vi "Main.vi"() -> ()   [LabVIEW 2016]
doc: "This template is for the Queued Message Handler design pattern.\n\nThe Event Handling Loop generates messages based on user interface actions.\n\nThe Message Handling Loop processes messages generated by the Event Handling Loop, or by other messages. The messages are string values, so new messages can be added easily to the Message Cases case structure in the Message Handling Loop. Each message cluster can also provide an optional value for Message Data, which is a variant that can be converted to whatever message-specific data is required."
uses:
  controls/UI Data.ctl
  support/Message Queue/Message Queue.lvlib
  <vilib>/Utility/error.llb/Error Cluster From Error Code.vi
  support/User Event - Stop/User Event - Stop.lvlib
  support/Message Queue/Enqueue Message (Single).vi
  <vilib>/ErrorRing/Error Ring.xnode
  <vilib>/SmarAct/MCS/Types/mcsSensorTypes.ctl
  helper/revolution_parameters.ctl
panel:
  in  "revolution":i32
  in  "Init Stages":bool
  out "stepsize y":dbl
  out "stepsize x":dbl
  in  "Iteration":u32=1
  in  "RESET PREV RUN":bool
  in  "ABORT":bool
  in  "RUN TABLE":bool
  in  "Angle":i32=16960
  in  "DISTANCE Y":i32=16960
  in  "one revolution":bool
  in  "steps Y":i32
  in  "scan length y (micron)":dbl format="%#_13g"
  out "polling iteration":i32=3
  in  "System locator":string(combo)="usb:id:425839965"
  in  "findSystems":bool caption="Find Systems"
  out "hw loop current msg":string="Exit"
  in  "init loops test":bool
  in  "stop":bool
  in  "DISTANCE X":i32=16960
  in  "one step y":bool
  in  "one step x":bool
  out "channelIndex":u32
  out "data1 2":u32=143
  out "packetType":T1(ring)=enum."SA_ERROR_ PACKET_TYPE"
  in  "connect":bool
  out "connected":bool=TRUE
  in  "Amplitude":u32=4000 min=1 max=4000 step=1
  in  "Frequency":u32=8000 min=1 max=18500 step=1
  in  "Rotation channel":u32
  in  "Y channel":u32=2
  out "Error":errorcluster
  in  "X channel":u32=1
  out "System Index":u32=35
  out "Y array":dbl[](array[numeric])
  out "X array":dbl[](array[numeric])
  in  "scan length x (micron)":dbl format="%#_13g"
  in  "steps X":i32
  in  "calc table":bool=TRUE
  in  "Home":bool
  out "Display <Replace Me>":string="\"Exit\" button pressed"
  in  "Do Something Else <Replace Me>":bool
  in  "Do Something <Replace Me>":bool
  in  "Exit":bool
  # "These controls have associated \"Value Changed\" events configured in the Event Structure on the diagram.\n\nReplace them (and reconfigure the Event Structure) with the controls you need for your application."
  # "This template is for the Queued Message Handler design pattern.\n\nSee the block diagram for more information on how to use this template."
  # "POLLING"
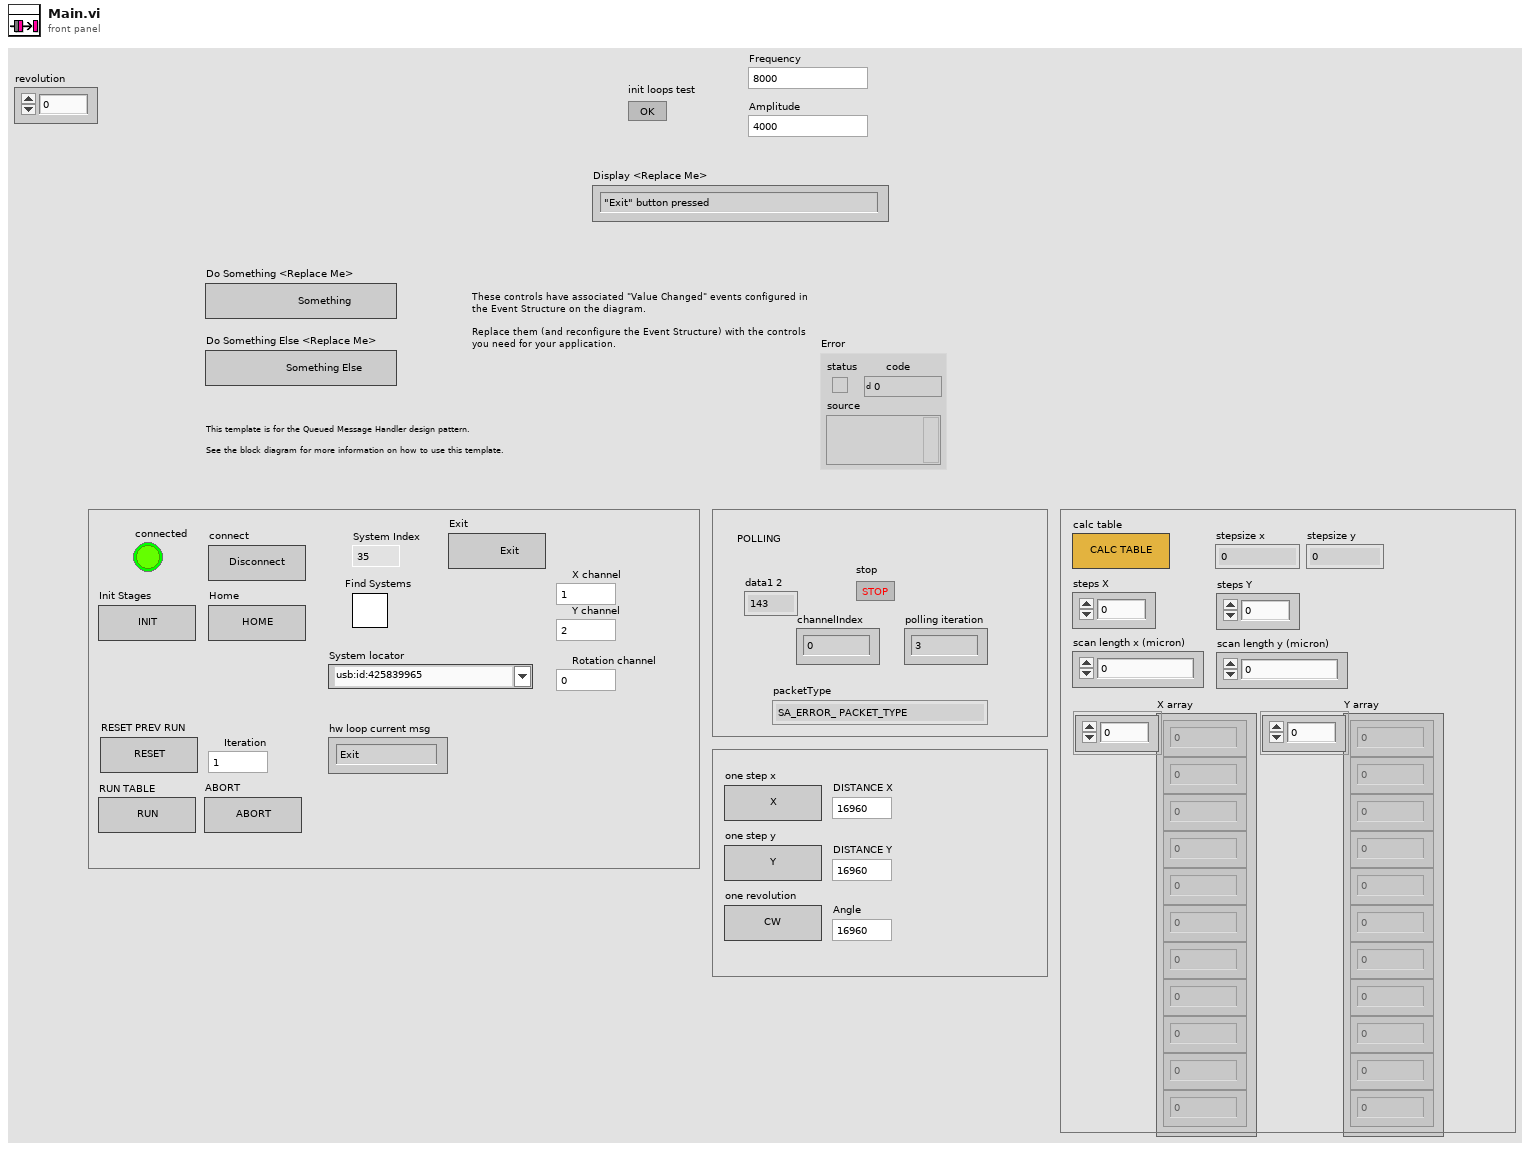
[diagram p1: front panel]
types:
  T1 = enum32{"SA_NO PACKET_TYPE", "SA_ERROR_ PACKET_TYPE", "SA_POSITION PACKET_TYPE", "SA_COMPLETED PACKET_TYPE", "SA_STATUS PACKET_TYPE", "SA_ANGLE_PACKET_TYPE", "SA_VOLTAGE_LEVEL_PACKET_TYPE", "SA_SENSOR_TYPE_PACKET_TYPE", "SA_SENSOR_ENABLED_PACKET_TYPE", "SA_END_EFFECTOR_TYPE_PACKET_TYPE", "SA_GRIPPER_OPENING_PACKET_TYPE", "SA_FORCE_PACKET_TYPE", "SA_MOVE_SPEED_PACKET_TYPE", "SA_PHYSICAL_POSITION_KNOWN_PACKET_TYPE", "SA_POSITION_LIMIT_PACKET_TYPE", "SA_ANGLE_LIMIT_PACKET_TYPE", "SA_SAFE_DIRECTION_PACKET_TYPE", "SA_SCALE_PACKET_TYPE", "SA_MOVE_ACCELERATION_PACKET_TYPE", "SA_CHANNEL_PROPERTY_PACKET_TYPE", "SA_CAPTURE_BUFFER_PACKET_TYPE", "SA_TRIGGERED_PACKET_TYPE"}
  T2 = typedef "UI Data.ctl" = cluster{"Boolean <Replace Me>":bool, "String <Replace Me>":string, "Numeric <Replace Me>":dbl, "Do Something Ref":refnum<vi>, "Do Something Else Ref":refnum<vi>, "Data Display Ref":refnum<vi>, "Exit Button Ref":refnum<vi>}
  T3 = typedef "Message Queue.lvlib/All Message Queues.ctl" = cluster{"UI":refnum<queue>, "queue out":refnum<queue>}
  T4 = typedef "mcsSensorTypes.ctl" = enum32{"SA_NO_SENSOR_TYPE", "SA_S_SENSOR_TYPE", "SA_SR_SENSOR_TYPE", "SA_ML_SENSOR_TYPE", "SA_MR_SENSOR_TYPE", "SA_SP_SENSOR_TYPE", "SA_SC_SENSOR_TYPE", "SA_M25_SENSOR_TYPE", "SA_SR20_SENSOR_TYPE", "SA_M_SENSOR_TYPE", "SA_GC_SENSOR_TYPE", "SA_GD_SENSOR_TYPE", "SA_GE_SENSOR_TYPE", "SA_RA_SENSOR_TYPE", "SA_GF_SENSOR_TYPE", "SA_RB_SENSOR_TYPE", "SA_G605S_SENSOR_TYPE", "SA_G775S_SENSOR_TYPE", "SA_SC500_SENSOR_TYPE", "SA_G955S_SENSOR_TYPE", "SA_SR77_SENSOR_TYPE", "SA_SD_SENSOR_TYPE", "SA_R20ME_SENSOR_TYPE", "SA_SR2_SENSOR_TYPE", "SA_SCD_SENSOR_TYPE", "SA_SRC_SENSOR_TYPE", "SA_SR36M_SENSOR_TYPE", "SA_SR36ME_SENSOR_TYPE", "SA_SR50M_SENSOR_TYPE", "SA_SR50ME_SENSOR_TYPE", "SA_G1045S_SENSOR_TYPE", "SA_G1395S_SENSOR_TYPE", "SA_MD_SENSOR_TYPE", "SA_G935M_SENSOR_TYPE", "SA_SHL20_SENSOR_TYPE", "SA_SCT_SENSOR_TYPE", "SA_SR77T_SENSOR_TYPE", "SA_SR120_SENSOR_TYPE", "SA_LC_SENSOR_TYPE", "SA_LR_SENSOR_TYPE", "SA_LCD_SENSOR_TYPE", "SA_L_SENSOR_TYPE", "SA_LD_SENSOR_TYPE", "SA_LE_SENSOR_TYPE", "SA_LED_SENSOR_TYPE", "SA_GDD_SENSOR_TYPE", "SA_GED_SENSOR_TYPE", "SA_G935S_SENSOR_TYPE", "SA_G605DS_SENSOR_TYPE", "SA_G775DS_SENSOR_TYPE"}
  T5 = enum32{"SA_NO_REPORT_ON_COMPLETE", "SA_REPORT_ON_COMPLETE"}
  T6 = enum32{"SA_SENSOR_DISABLED", "SA_SENSOR_ENABLED", "SA_SENSOR_POWERSAVE"}
  T7 = enum32{"SA_UNBUFFERED_OUTPUT", "SA_BUFFERED_OUTPUT"}
  T8 = typedef "revolution_parameters.ctl" = cluster{"revolution":i32, "angle":i32}
  T9 = typedef "mcsPacket.ctl" = cluster{"packetType":enum32{"SA_NO PACKET_TYPE", "SA_ERROR_ PACKET_TYPE", "SA_POSITION PACKET_TYPE", "SA_COMPLETED PACKET_TYPE", "SA_STATUS PACKET_TYPE", "SA_ANGLE_PACKET_TYPE", "SA_VOLTAGE_LEVEL_PACKET_TYPE", "SA_SENSOR_TYPE_PACKET_TYPE", "SA_SENSOR_ENABLED_PACKET_TYPE", "SA_END_EFFECTOR_TYPE_PACKET_TYPE", "SA_GRIPPER_OPENING_PACKET_TYPE", "SA_FORCE_PACKET_TYPE", "SA_MOVE_SPEED_PACKET_TYPE", "SA_PHYSICAL_POSITION_KNOWN_PACKET_TYPE", "SA_POSITION_LIMIT_PACKET_TYPE", "SA_ANGLE_LIMIT_PACKET_TYPE", "SA_SAFE_DIRECTION_PACKET_TYPE", "SA_SCALE_PACKET_TYPE", "SA_MOVE_ACCELERATION_PACKET_TYPE", "SA_CHANNEL_PROPERTY_PACKET_TYPE", "SA_CAPTURE_BUFFER_PACKET_TYPE", "SA_TRIGGERED_PACKET_TYPE"}, "channelIndex":u32, "data1":u32, "data2":i32, "data3":i32, "data4":u32}
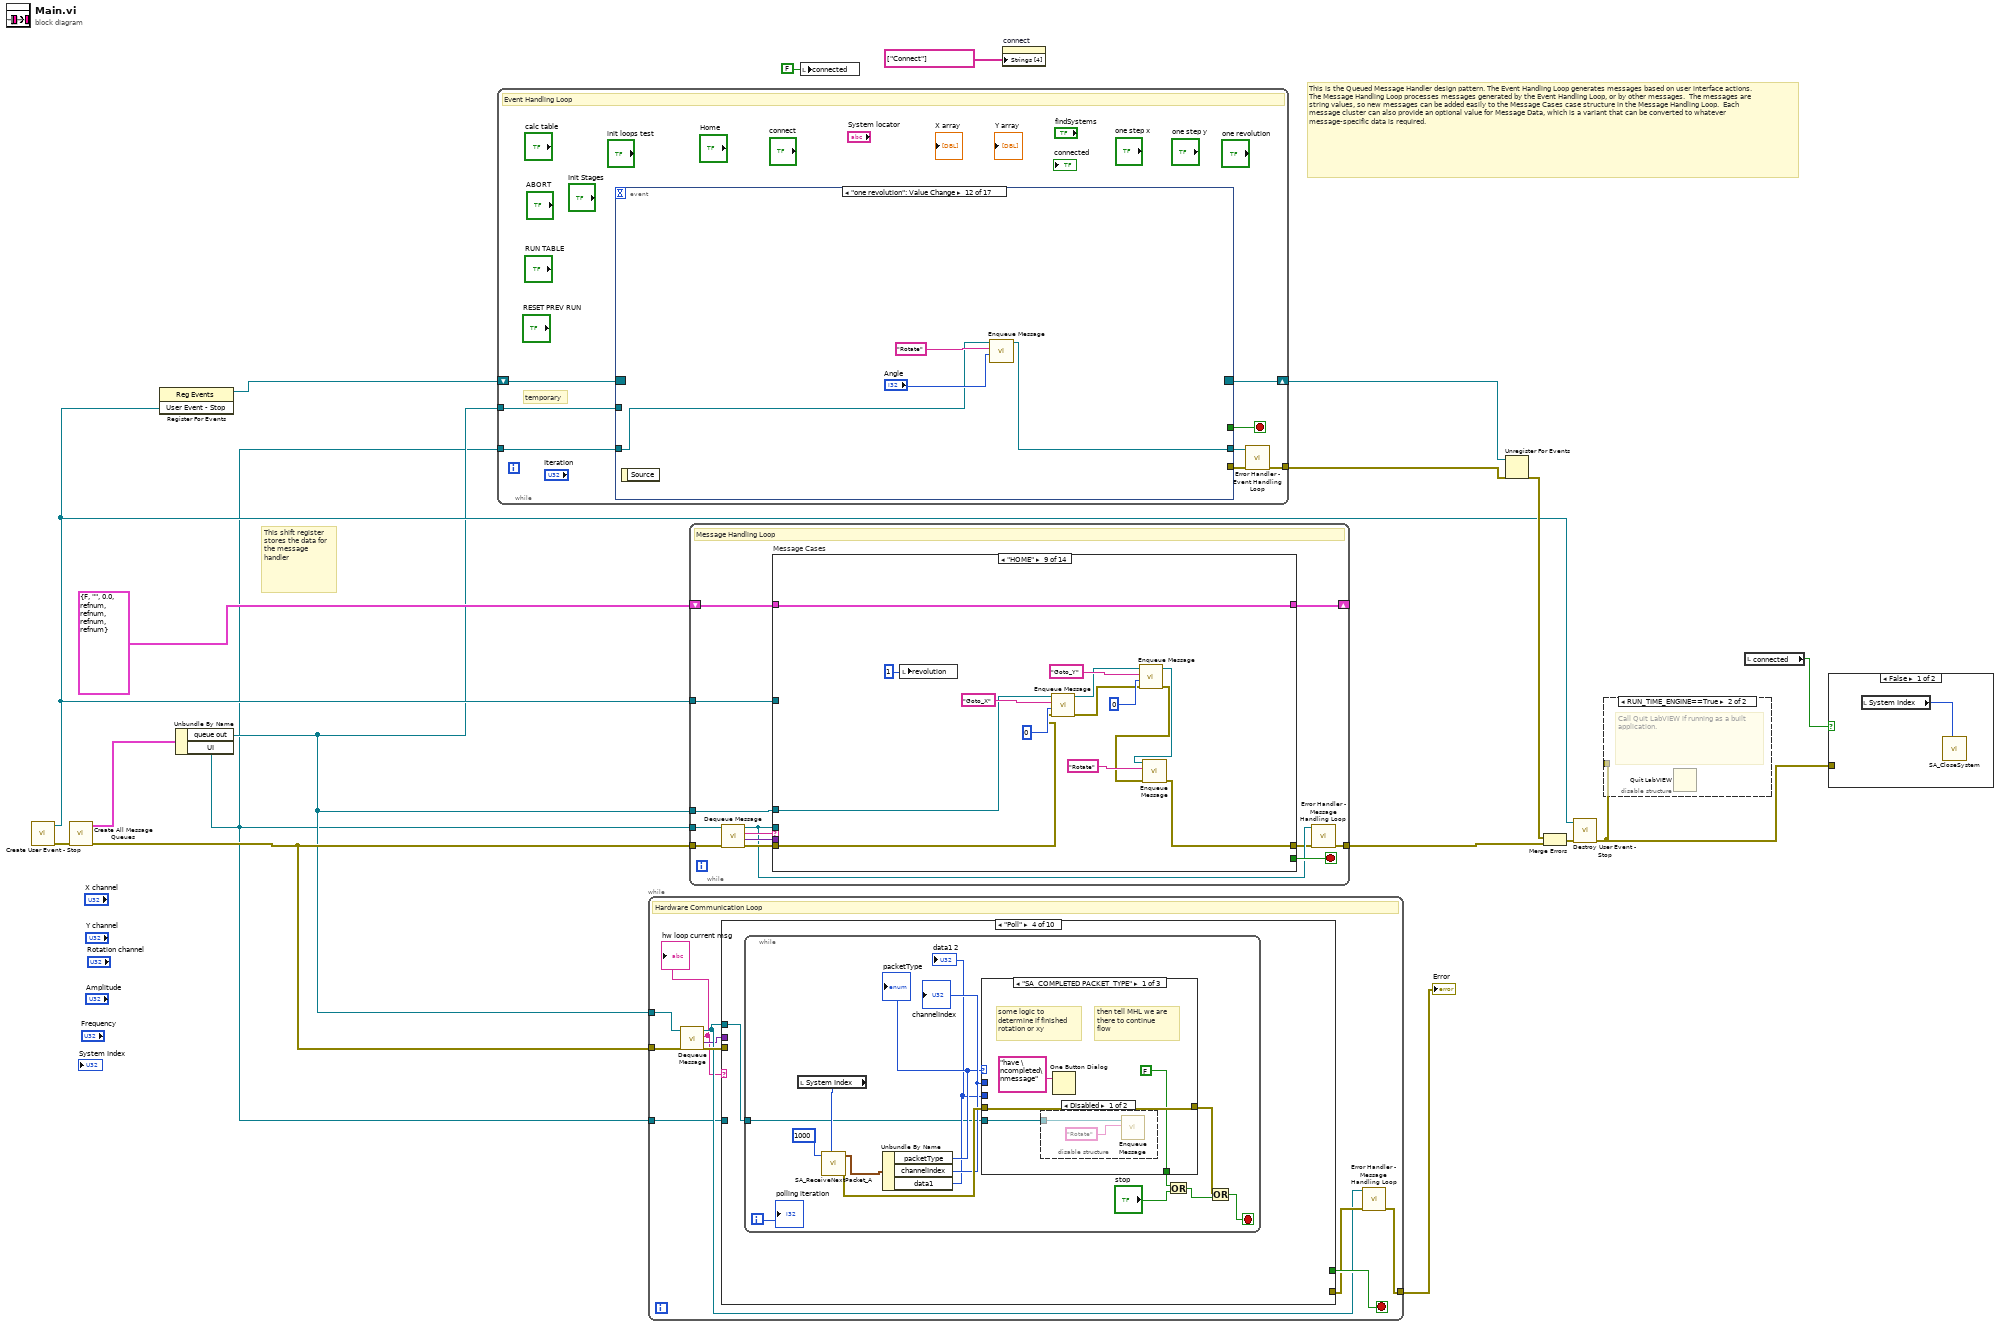
[diagram p0: block diagram]
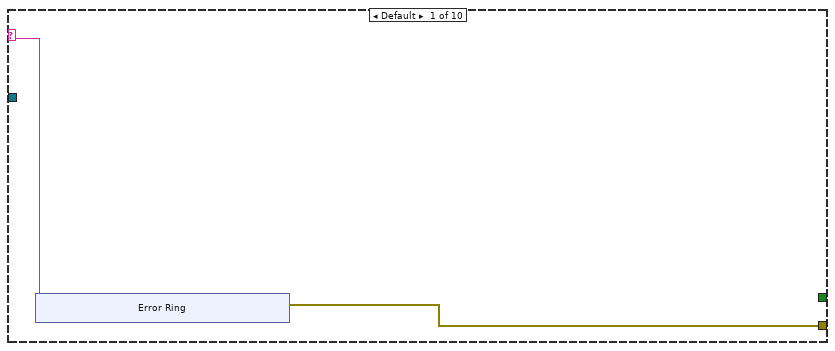
[diagram p3: hidden frame]
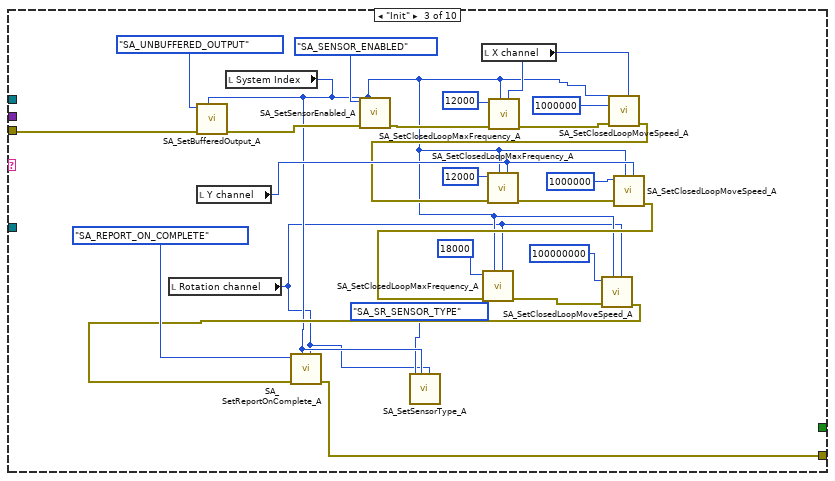
[diagram p5: hidden frame]
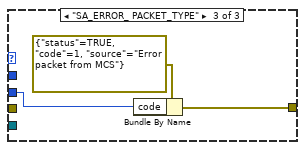
[diagram p8: hidden frame]
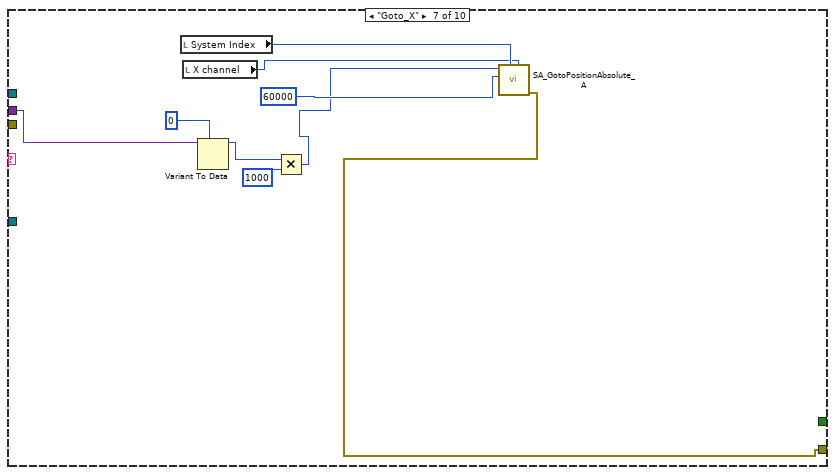
[diagram p11: hidden frame]
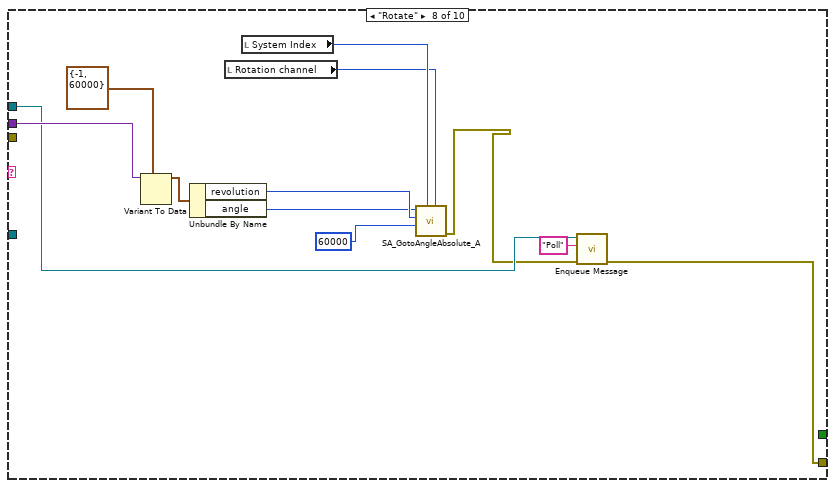
[diagram p12: hidden frame]
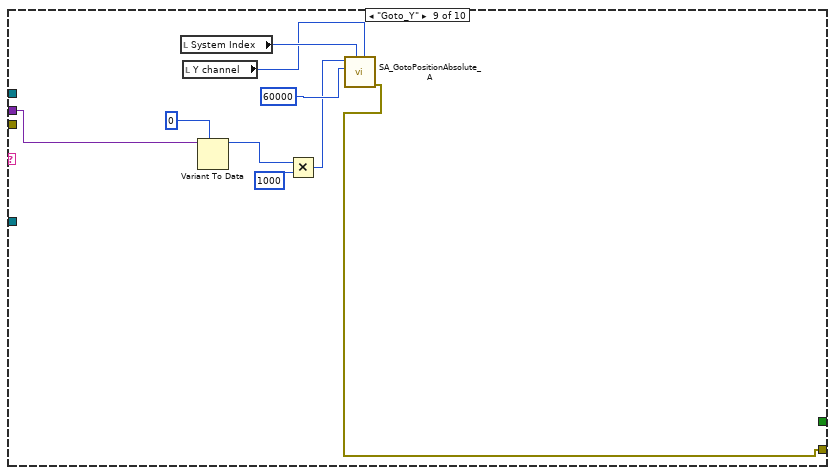
[diagram p13: hidden frame]
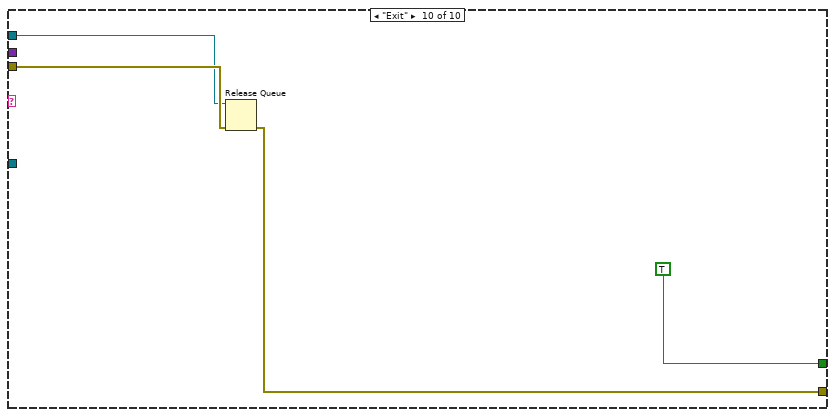
[diagram p14: hidden frame]
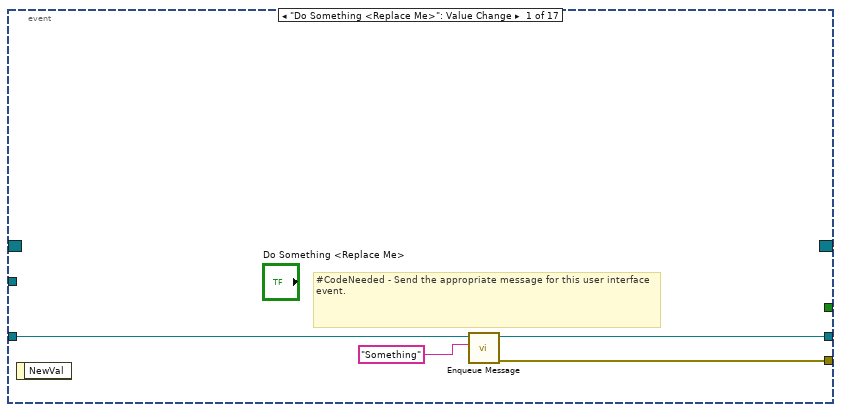
[diagram p16: hidden frame]
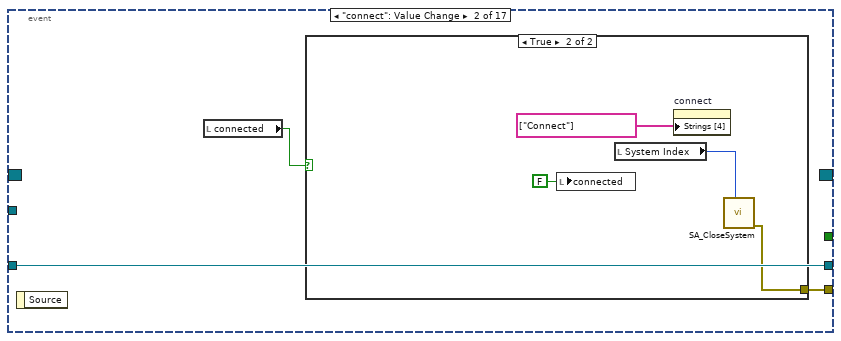
[diagram p17: hidden frame]
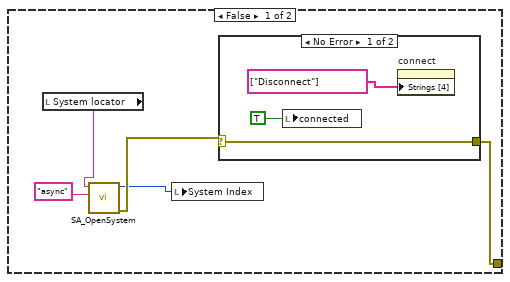
[diagram p18: hidden frame]
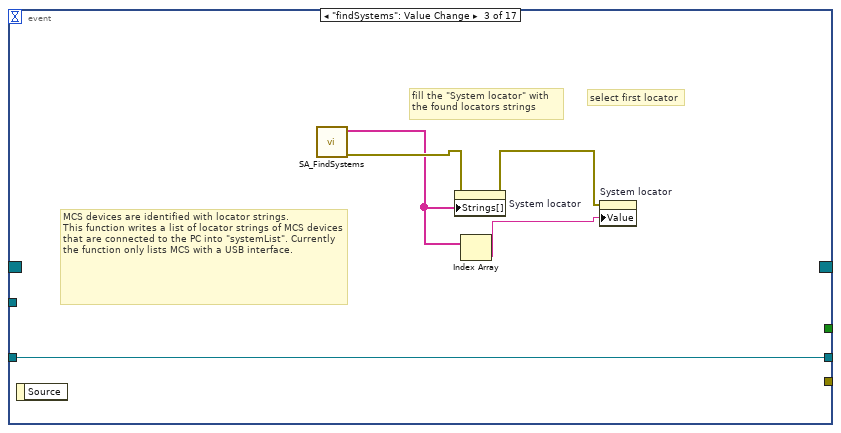
[diagram p20: hidden frame]
diagram:
  # "This is the Queued Message Handler design pattern. The Event Handling Loop generates messages based on user interface actions. The Message Handling Loop processes messages generated by the Event Handling Loop, or by other messages.  The messages are string values, so new messages can be added easily to the Message Cases case structure in the Message Handling Loop.  Each message cluster can also provide an optional value for Message Data, which is a variant that can be converted to whatever message-specific data is required."
  # "This shift register stores the data for the message handler"
  n1 = call "Create User Event - Stop.vi"() -> ("error out"=w16:errorcluster, "User Event - Stop"=w9:refnum<user-event>)  [unwired: 10 in]
  n2 = call "Create All Message Queues.vi"("error in (no error)"=w16) -> ("error out"=w7:errorcluster, "Message Queues out"=w18:T3)  [unwired: 9 in]
  n3 = register-events(w9) -> (reference out=w10:refnum<event-registration>)  [unwired: 2 in, 1 out]
  n4 = Unbundle By Name(w18) -> ("queue out"=w2:refnum<queue>, "UI"=w1:refnum<queue>)
  n5 = while {
    tunnel: w1 -> [w26]
    shift-right: [w24] -> w13
    shift-left: w10 -> [w25]
    tunnel: [w20] -> w11
    tunnel: w2 -> [w19]
    stop <- w22 stop-if-true
    # "temporary"
    # "Event Handling Loop"
    n6 = event shown="[11] \"one revolution\": Value Change" {
      selector: w25 -> [_ _ _ _ _ _ _ _ _ _ _ _ _ _ _ _ _]
      dyn-events: [_ _ _ _ _ _ _ _ _ _ _ _ _ _ _ _ _] -> w24
      timeout: _ -> [_ _ _ _ _ _ _ _ _ _ _ _ _ _ _ _ _]
      tunnel: [_ _ _ _ _ _ _ _ _ _ _ _ _ _ _ _ TRUE ("Discard?")] -> w22
      tunnel: w26 -> [w30 w33 w51 w55 w57 w66 w70 w72 w77 w78 w83 w87 w93 w98 w100 w105 w108]
      tunnel: [w27 w32 _ w52 _ _ w68 _ w75 _ _ _ w90 w97 _ w104 _] -> w23
      tunnel: [w29 w33 w51 w54 w57 w66 w69 w71 w76 w78 w83 w86 w92 w96 w100 w103 w108] -> w21
      tunnel: w19 -> [_ _ _ _ _ _ _ _ _ w79 w84 _ _ _ _ _ _]
      event "Do Something <Replace Me>": Value Change {
        # "#CodeNeeded - Send the appropriate message for this user interface event."
        n7 = event-data() -> ()  [unwired: 1 in, 1 out]
        n8 = call-poly "Enqueue Message.vi"("Message"="Something", "Message Queue"=w30) -> ("error out"=w27:errorcluster, "dup Message Queue"=w29:refnum<queue>)  [unwired: 8 in]
      }
      event "connect": Value Change {
        n9 = event-data() -> ()  [unwired: 1 in, 1 out]
        n10 = local read "connected"() -> (w31:bool)
        n11 = case shown="True" w31 {
          tunnel: [w36 w43] -> w32
          frame False {
            n12 = local read "System locator"() -> (w35:string)
            n13 = call <vilib>:"SA_OpenSystem.vi"("options"="async", "systemLocator"=w35) -> ("error out"=w37:errorcluster, "systemIndexOut"=w34:u32)  [unwired: 8 in]
            n14 = local write "System Index"(w34) -> ()
            n15 = case shown="No Error" w37 {
              selector: w37 -> [w40 w42]
              tunnel: [w40 w42] -> w36
              frame No Error {
                n16 = local write "connected"(TRUE ("connected")) -> ()
                n17 = property on="connect" class="Bool"("Strings [4]"=string[] ["Disconnect"]) -> ()  [unwired: 2 in, 2 out]
              }
              frame Error {
              }
            }
          }
          frame True {
            n18 = local write "connected"(FALSE ("connected")) -> ()
            n19 = local read "System Index"() -> (w44:u32)
            n20 = property on="connect" class="Bool"("Strings [4]"=string[] ["Connect"]) -> ()  [unwired: 2 in, 2 out]
            n21 = call <vilib>:"SA_CloseSystem.vi"("systemIndex"=w44) -> ("error out"=w43:errorcluster)  [unwired: 10 in]
          }
        }
      }
      event "findSystems": Value Change {
        # "select first locator"
        # "fill the \"System locator\" with\nthe found locators strings"
        # "MCS devices are identified with locator strings.\nThis function writes a list of locator strings of MCS devices that are connected to the PC into \"systemList\". Currently the function only lists MCS with a USB interface."
        n22 = event-data() -> ()  [unwired: 1 in, 1 out]
        n23 = call <vilib>:"SA_FindSystems.vi"() -> ("error out"=w50:errorcluster, "systemList"=w49:string[])  [unwired: 10 in]
        n24 = property on="System locator" class="CmbBox"(error in=w50, "Strings[]"=w49) -> (error out=w48:errorcluster)  [unwired: 1 in, 1 out]
        n25 = Index Array(array=w49) -> (element=w47:string)  [unwired: 1 in]
        n26 = property on="System locator" class="CmbBox"(error in=w48, "Value"=w47) -> ()  [unwired: 1 in, 2 out]
      }
      event "init loops test": Value Change {
        n27 = event-data() -> ()  [unwired: 1 in, 1 out]
        n28 = call-poly "Enqueue Message.vi"("Message"="initialize", "Message Queue"=w55) -> ("error out"=w52:errorcluster, "dup Message Queue"=w54:refnum<queue>)  [unwired: 8 in]
      }
      event "RESET PREV RUN": Value Change {
        n29 = event-data() -> ()  [unwired: 1 in, 1 out]
        n30 = local write "Iteration"(u32 0 ("Iteration")) -> ()
      }
      event "calc table": Value Change {
        # "these are both 1D arrays \nof length stepsx * stepsy\nessentially lookup tables"
        n31 = event-data() -> ()  [unwired: 1 in, 1 out]
        n32 = call "calculateTableSimpleSerpentine.vi"("scan length y"="scan length y (micron)", "steps Y"="steps Y", "scan length x"="scan length x (micron)", "steps X"="steps X") -> ("stepsize y"=→"stepsize y":dbl, "final array Y"=w60:dbl[], "stepsize x"=→"stepsize x":dbl, "final array X"=w61:dbl[])
        n33 = local write "Y array"(w60) -> ()
        n34 = local write "X array"(w61) -> ()
      }
      event "Home": Value Change {
        n35 = event-data() -> ()  [unwired: 1 in, 1 out]
        n36 = call-poly "Enqueue Message.vi"("Message"="HOME", "Message Queue"=w70) -> ("error out"=w68:errorcluster, "dup Message Queue"=w69:refnum<queue>)  [unwired: 8 in]
      }
      event "Init Stages": Value Change {
        n37 = event-data() -> ()  [unwired: 1 in, 1 out]
        n38 = call-poly "Enqueue Message.vi"("Message"="START", "Message Queue"=w72) -> ("dup Message Queue"=w71:refnum<queue>)  [unwired: 8 in, 1 out]
      }
      event "RUN TABLE": Value Change {
        n39 = event-data() -> ()  [unwired: 1 in, 1 out]
        n40 = call-poly "Enqueue Message.vi"("Message"="Move_XY", "Message Queue"=w77) -> ("error out"=w75:errorcluster, "dup Message Queue"=w76:refnum<queue>)  [unwired: 8 in]
      }
      event "one step x": Value Change {
        n41 = event-data() -> ()  [unwired: 1 in, 1 out]
        n42 = call-poly "Enqueue Message.vi"("Message Data"="DISTANCE X", "Message"="Goto_X", "Message Queue"=w79) -> ()  [unwired: 7 in, 2 out]
      }
      event "one step y": Value Change {
        n43 = event-data() -> ()  [unwired: 1 in, 1 out]
        n44 = call-poly "Enqueue Message.vi"("Message Data"="DISTANCE Y", "Message"="Goto_Y", "Message Queue"=w84) -> ()  [unwired: 7 in, 2 out]
      }
      event "one revolution": Value Change {
        n45 = event-data() -> ()  [unwired: 1 in, 1 out]
        n46 = call-poly "Enqueue Message.vi"("Message Data"="Angle", "Message"="Rotate", "Message Queue"=w87) -> ("dup Message Queue"=w86:refnum<queue>)  [unwired: 7 in, 1 out]
      }
      event "Do Something Else <Replace Me>": Value Change {
        # "#CodeNeeded - Send the appropriate message for this user interface event."
        n47 = event-data() -> ()  [unwired: 1 in, 1 out]
        n48 = call-poly "Enqueue Message.vi"("Message"="Something Else", "Message Queue"=w93) -> ("error out"=w90:errorcluster, "dup Message Queue"=w92:refnum<queue>)  [unwired: 8 in]
      }
      event Panel Close? {
        # "Send the 'Confirm Quit' message if the user closes the panel of the VI. Discard the event so the 'Confirm Quit' message has a chance to run."
        n49 = event-data() -> ()  [unwired: 1 in, 1 out]
        n50 = call-poly "Enqueue Message.vi"("Priority Message? (F)"=TRUE, "Message"="Confirm Quit", "Message Queue"=w98) -> ("error out"=w97:errorcluster, "dup Message Queue"=w96:refnum<queue>)  [unwired: 7 in]
        n51 = event-data("Discard?"=TRUE) -> ()  [unwired: 1 in, 1 out]
      }
      event Application Instance Close {
        # "#CodeRecommended - When a project closes, all VIs within that project are aborted and leave memory. However, any code placed in this event frame is guaranteed to run to completion, so add any cleanup code that absolutely must happen here."
        n52 = event-data() -> ()  [unwired: 1 in, 1 out]
      }
      event "Exit": Value Change {
        n53 = event-data() -> ()  [unwired: 1 in, 1 out]
        n54 = call-poly "Enqueue Message.vi"("Priority Message? (F)"=TRUE, "Message"="Exit", "Message Queue"=w105) -> ("error out"=w104:errorcluster, "dup Message Queue"=w103:refnum<queue>)  [unwired: 7 in]
      }
      event User Event {
        # "The Message Handling Loop processed an \"Exit\" message, which fired this event to stop the Event Handling Loop."
        n55 = event-data() -> ()  [unwired: 1 in, 1 out]
        n56 = local write "Display <Replace Me>"("\"Exit\" button pressed" ("VI Stopped")) -> ()
      }
    }
    n57 = call "Error Handler - Event Handling Loop.vi"("error in (no error)"=w23, "Message Queue"=w21) -> ("dup error in"=w20:errorcluster)  [unwired: 8 in, 1 out]
  }
  n58 = while {
    tunnel: w2 -> [w118]
    tunnel: [w114] -> w8
    tunnel: w7 -> [w111]
    tunnel: w1 -> [w109]
    stop <- w117 stop-if-true
    # "Hardware Communication Loop"
    n59 = call "Dequeue Message.vi"("error in (no error)"=w111, "Message Queue"=w118) -> ("error out"=w116:errorcluster, "Message Data"=w112:variant, "Message"=w110:string, "dup Message Queue"=w113:refnum<queue>)  [unwired: 6 in]
    "hw loop current msg" <- w110
    n60 = case shown="\"Poll\"" w110 {
      selector: w110 -> [w120 _ _ _ _ _ _ _ _ _]
      tunnel: [w119 _ w131 _ _ _ w180 w186 w204 w208] -> w115
      tunnel: [_ _ _ _ _ _ _ _ _ TRUE] -> w117
      tunnel: w116 -> [_ _ w135 _ _ _ _ _ _ w209]
      tunnel: w113 -> [_ _ _ w152 _ _ _ w189 _ w207]
      tunnel: w112 -> [_ _ _ _ _ _ w184 w197 w205 _]
      tunnel: w109 -> [_ _ _ _ _ _ _ _ _ _]
      frame Default {
        n61 = xnode "Error Ring"("parameter 0"=w120) -> ("error out"=w119:errorcluster)
      }
      frame "Initialize" {
      }
      frame "Init" {
        n62 = local read "Rotation channel"() -> (w128:u32)
        n63 = local read "Y channel"() -> (w140:u32)
        n64 = local read "System Index"() -> (w130:u32)
        n65 = call <vilib>:"SA_SetBufferedOutput_A.vi"("systemIndex"=w130, "error in (no error)"=w135, "mode"=T7."SA_UNBUFFERED_OUTPUT") -> ("error out"=w136:errorcluster)  [unwired: 8 in]
        n66 = call <vilib>:"SA_SetSensorEnabled_A.vi"("systemIndex"=w130, "error in (no error)"=w136, "enabled"=T6."SA_SENSOR_ENABLED") -> ("error out"=w139:errorcluster)  [unwired: 8 in]
        n67 = call <vilib>:"SA_SetSensorType_A.vi"("channelIndex"=w128, "systemIndex"=w130, "type"=mcsSensorTypes."SA_SR_SENSOR_TYPE") -> ()  [unwired: 8 in, 1 out]
        n68 = local read "X channel"() -> (w149:u32)
        n69 = call <vilib>:"SA_SetClosedLoopMaxFrequency_A.vi"("channelIndex"=w149, "systemIndex"=w130, "error in (no error)"=w139, "frequency"=u32 12000) -> ("error out"=w147:errorcluster)  [unwired: 7 in]
        n70 = call <vilib>:"SA_SetClosedLoopMoveSpeed_A.vi"("channelIndex"=w149, "systemIndex"=w130, "error in (no error)"=w147, "speed"=u32 1000000) -> ("error out"=w134:errorcluster)  [unwired: 7 in]
        n71 = call <vilib>:"SA_SetClosedLoopMaxFrequency_A.vi"("channelIndex"=w140, "systemIndex"=w130, "error in (no error)"=w134, "frequency"=u32 12000) -> ("error out"=w150:errorcluster)  [unwired: 7 in]
        n72 = call <vilib>:"SA_SetClosedLoopMoveSpeed_A.vi"("channelIndex"=w140, "systemIndex"=w130, "error in (no error)"=w150, "speed"=u32 1000000) -> ("error out"=w133:errorcluster)  [unwired: 7 in]
        n73 = call <vilib>:"SA_SetClosedLoopMaxFrequency_A.vi"("channelIndex"=w128, "systemIndex"=w130, "error in (no error)"=w133, "frequency"=u32 18000) -> ("error out"=w151:errorcluster)  [unwired: 7 in]
        n74 = call <vilib>:"SA_SetClosedLoopMoveSpeed_A.vi"("channelIndex"=w128, "systemIndex"=w130, "error in (no error)"=w151, "speed"=u32 100000000) -> ("error out"=w132:errorcluster)  [unwired: 7 in]
        n75 = call <vilib>:"SA_SetReportOnComplete_A.vi"("channelIndex"=w128, "systemIndex"=w130, "error in (no error)"=w132, "report"=T5."SA_REPORT_ON_COMPLETE") -> ("error out"=w131:errorcluster)  [unwired: 7 in]
      }
      frame "Poll" {
        n76 = while {
          tunnel: w152 -> [w156]
          i -> [w157]
          stop <- w159 stop-if-true
          n77 = local read "System Index"() -> (w161:u32)
          n78 = call <vilib>:"SA_ReceiveNextPacket_A.vi"("systemIndex"=w161, "timeout"=u32 1000) -> ("error out"=w166:errorcluster, "packet"=w163:T9)  [unwired: 8 in]
          n79 = Unbundle By Name(w163) -> ("packetType"=w164:T1, "channelIndex"=w165:u32, "data1"=w160:u32)
          "packetType" <- w164
          "channelIndex" <- w165
          "data1 2" <- w160
          n80 = case shown="\"SA_COMPLETED PACKET_TYPE\"" w164 {
            tunnel: [w170 w173 w175] -> w158
            tunnel: w160 -> [_ _ w174]
            tunnel: w165 -> [_ _ _]
            tunnel: w166 -> [w170 w173 _]
            tunnel: w156 -> [w168 _ _]
            tunnel: [FALSE ("x") _ _] -> w153
            frame "SA_COMPLETED PACKET_TYPE" {
              # "then tell MHL we are\nthere to continue\nflow"
              # "some logic to \ndetermine if finished\nrotation or xy"
              n81 = disable-structure shown="Disabled" {
                disable-tunnel: w168 -> [w171 _]
                frame Disabled {
                  n82 = call-poly "Enqueue Message.vi"("Message"="Rotate", "Message Queue"=w171) -> ()  [unwired: 8 in, 2 out]
                }
                frame Enabled {
                }
              }
              n83 = One Button Dialog(message="have \ncompleted\nmessage") -> ()  [unwired: 1 in, 1 out]
            }
            frame "SA_NO PACKET_TYPE", Default {
            }
            frame "SA_ERROR_ PACKET_TYPE" {
              n84 = Bundle By Name(cluster=errorcluster {"status"=TRUE, "code"=1, "source"="Error packet from MCS"} ("error out"), "code"=w174) -> (w175:errorcluster)
            }
          }
          n85 = Or(x=w153, y="stop") -> (x .or. y?=w154:bool)
          n86 = Or(x=w158, y=w154) -> (x .or. y?=w159:bool)
          "polling iteration" <- w157
        }
      }
      frame "Disable_guns" {
        # "send TTL signal"
      }
      frame "Enable_guns" {
        # "send TTL signal"
      }
      frame "Goto_X" {
        n87 = local read "System Index"() -> (w182:u32)
        n88 = local read "X channel"() -> (w181:u32)
        n89 = Variant To Data(type=0 ("DISTANCE X 2"), Variant=w184) -> (data=w179:i32)  [unwired: 1 in, 1 out]
        n90 = Multiply(x=w179, y=1000) -> (x*y=w178:i32)
        n91 = call <vilib>:"SA_GotoPositionAbsolute_A.vi"("channelIndex"=w181, "systemIndex"=w182, "holdTime"=u32 60000, "position"=w178) -> ("error out"=w180:errorcluster)  [unwired: 7 in]
      }
      frame "Rotate" {
        n92 = Variant To Data(type=T8 {"revolution"=-1, "angle"=60000} ("Cluster"), Variant=w197) -> (data=w192:T8)  [unwired: 1 in, 1 out]
        n93 = Unbundle By Name(w192) -> ("revolution"=w191:i32, "angle"=w190:i32)
        n94 = local read "Rotation channel"() -> (w195:u32)
        n95 = local read "System Index"() -> (w196:u32)
        n96 = call <vilib>:"SA_GotoAngleAbsolute_A.vi"("channelIndex"=w195, "systemIndex"=w196, "holdTime"=u32 60000, "revolution"=w191, "angle"=w190) -> ("error out"=w187:errorcluster)  [unwired: 6 in]
        n97 = call-poly "Enqueue Message.vi"("error in (no error)"=w187, "Message"="Poll", "Message Queue"=w189) -> ("error out"=w186:errorcluster)  [unwired: 7 in, 1 out]
      }
      frame "Goto_Y" {
        n98 = local read "System Index"() -> (w202:u32)
        n99 = local read "Y channel"() -> (w201:u32)
        n100 = Variant To Data(type=0 ("DISTANCE X 2"), Variant=w205) -> (data=w199:i32)  [unwired: 1 in, 1 out]
        n101 = Multiply(x=w199, y=1000) -> (x*y=w198:i32)
        n102 = call <vilib>:"SA_GotoPositionAbsolute_A.vi"("channelIndex"=w201, "systemIndex"=w202, "holdTime"=u32 60000, "position"=w198) -> ("error out"=w204:errorcluster)  [unwired: 7 in]
      }
      frame "Exit" {
        n103 = Release Queue(queue=w207, error in (no error)=w209) -> (error out=w208:errorcluster)  [unwired: 1 in, 2 out]
      }
    }
    n104 = call "Error Handler - Message Handling Loop.vi"("error in (no error)"=w115, "Message Queue"=w113) -> ("dup error in"=w114:errorcluster)  [unwired: 8 in, 1 out]
  }
  "Error" <- w8
  n105 = while {
    tunnel: w1 -> [w216]
    shift-right: [w223] -> _
    shift-left: T2 {"Boolean <Replace Me>"=FALSE, "String <Replace Me>"="", "Numeric <Replace Me>"=0.0, "Do Something Ref"=refnum, "Do Something Else Ref"=refnum, "Data Display Ref"=refnum, "Exit Button Ref"=refnum} ("Data Cluster") -> [w211]
    tunnel: w9 -> [w221]
    tunnel: w7 -> [w220]
    tunnel: [w214] -> w17
    tunnel: w2 -> [w212]
    stop <- w222 stop-if-true
    # "Message Handling Loop"
    n106 = call "Dequeue Message.vi"("error in (no error)"=w220, "Message Queue"=w216) -> ("error out"=w219:errorcluster, "Message Data"=w217:variant, "Message"=w218:string, "dup Message Queue"=w215:refnum<queue>)  [unwired: 6 in]
    n107 = case "Message Cases" shown="\"HOME\"" w218 {
      selector: w218 -> [_ _ _ _ _ _ _ _ _ _ _ _ _ w335]
      tunnel: w215 -> [w225 w237 w244 _ _ w265 _ _ _ w294 _ _ w334 _]
      tunnel: w219 -> [w233 w239 w246 w253 w262 w269 w272 w275 w284 w305 w316 w320 w327 _]
      tunnel: [w234 w240 w247 w254 w256 w267 w270 w276 w279 w306 w316 w320 w330 w336] -> w213
      tunnel: w211 -> [w232 w241 w248 w255 w261 w268 w271 w277 w291 w307 w315 w319 w333 w337]
      tunnel: [w231 w241 w248 w255 w261 w268 w271 w277 w291 w307 w315 w319 w333 w337] -> w223
      tunnel: [_ _ _ _ _ _ _ _ _ _ _ _ TRUE _] -> w222
      tunnel: w217 -> [_ _ _ w252 w260 _ _ _ _ _ _ _ w324 _]
      tunnel: w221 -> [_ _ _ _ _ _ _ _ _ _ _ _ w329 _]
      tunnel: w212 -> [_ _ _ _ _ _ _ w274 w289 w297 w313 _ w323 _]
      frame "Initialize" {
        w224 = "Initial Message" ("Initial Message")
        # "Bundle control references and a sample string value."
        # "Initialize - All initialization work should take place in this message, since other loops can potentially enqueue messages that execute immediately after this one."
        n108 = control-ref of="Do Something <Replace Me>"() -> (w230:refnum<vi>)
        n109 = control-ref of="Do Something Else <Replace Me>"() -> (w229:refnum<vi>)
        n110 = control-ref of="Exit"() -> (w227:refnum<vi>)
        n111 = control-ref of="Display <Replace Me>"() -> (w228:refnum<vi>)
        n112 = Bundle By Name(cluster=w232, "Do Something Ref"=w230, "Do Something Else Ref"=w229, "Data Display Ref"=w228, "Exit Button Ref"=w227, "String <Replace Me>"=w224) -> (w231:T2)
        n113 = call-poly "Enqueue Message.vi"("error in (no error)"=w233, "Message Data"=w224, "Message"="Update Display", "Message Queue"=w225) -> ("error out"=w234:errorcluster)  [unwired: 6 in, 1 out]
      }
      frame "Something" {
        # "Send string to \"Update Display\" message"
        # "#CodeNeeded - Perform whatever actions correspond to the \"Something\" message."
        # "Something - Replace this message with functionality for your own application."
        n114 = call-poly "Enqueue Message.vi"("error in (no error)"=w239, "Message Data"="\"Do Something\" button pressed" ("\"Do Something\" button pressed"), "Message"="Update Display", "Message Queue"=w237) -> ("error out"=w238:errorcluster)  [unwired: 6 in, 1 out]
        n115 = Merge Errors(w238) -> (w240:errorcluster)
      }
      frame "Something Else" {
        # "Send string to \"Update Display\" message"
        # "#CodeNeeded - Perform whatever actions correspond to the \"Something Else\" message."
        # "Something Else - Replace this message with functionality for your own application."
        n116 = call-poly "Enqueue Message.vi"("error in (no error)"=w246, "Message Data"="\"Do Something Else\" button pressed" ("\"Do Something Else\" button pressed"), "Message"="Update Display", "Message Queue"=w244) -> ("error out"=w245:errorcluster)  [unwired: 6 in, 1 out]
        n117 = Merge Errors(w245) -> (w247:errorcluster)
      }
      frame "Update Display" {
        # "#CodeRecommended - If you wish to decouple the Message Handling Loop from your user interface, consider creating User Events (like the \"Stop\" event in this VI) to message the Event Handling Loop whenever the user interface needs updating."
        # "Update Display - Convert the message data to a string to display in the Data Display indicator."
        n118 = Variant To Data(error in=w253, type="", Variant=w252) -> (data=→"Display <Replace Me>":string, error out=w250:errorcluster)
        n119 = Merge Errors(w250) -> (w254:errorcluster)
      }
      frame "Error" {
        # "#CodeRecommended - If you ever change the name of this \"Error\" message, you'll need to update the name in the Check Loop Error.vi as well."
        # "#CodeRecommended - Consider creating a system for logging errors in some way. These errors are for notification purposes only. Handling of specific errors should be performed in the message frames that generated the error."
        # "Error - Display an error dialog. This message is sent by the \"Error Handler\" VIs at the end of other loops in this application."
        n120 = Variant To Data(error in=w262, type=errorcluster {"status"=FALSE, "code"=0, "source"=""} ("error constant"), Variant=w260) -> (data=w258:errorcluster, error out=w257:errorcluster)
        n121 = call <vilib>:"Simple Error Handler.vi"("error in (no error)"=w258) -> ()  [unwired: 4 in, 5 out]
        n122 = Merge Errors(w257) -> (w256:errorcluster)
      }
      frame "Confirm Quit" {
        # "#CodeNeeded - If you want to provide an \"Are you sure\" dialog (or some other notification) before the application exits, place that code here. This message is typically sent from a Panel Close? event."
        # "Confirm Quit - Message that can confirm whether or not the user wants to exit the application."
        n123 = call-poly "Enqueue Message.vi"("Priority Message? (F)"=TRUE, "error in (no error)"=w269, "Message"="Exit", "Message Queue"=w265) -> ("error out"=w266:errorcluster)  [unwired: 6 in, 1 out]
        n124 = Merge Errors(w266) -> (w267:errorcluster)
      }
      frame "---Copy This Frame---" {
        # "Duplicate this frame when creating new messages.  Change this comment in the duplicated frame to describe this message."
        n125 = Merge Errors(w272) -> (w270:errorcluster)
      }
      frame "START" {
        # "init HW loop communication/parameters"
        # "iterate through matrix"
        n126 = call-poly "Enqueue Message.vi"("Message"="Init", "Message Queue"=w274) -> ()  [unwired: 8 in, 2 out]
        n127 = Merge Errors(w275) -> (w276:errorcluster)
      }
      frame "HOME" {
        n128 = local write "revolution"(1 ("revolution")) -> ()
        n129 = call-poly "Enqueue Message.vi"("error in (no error)"=w284, "Message Data"=0 ("DISTANCE X 2"), "Message"="Goto_X", "Message Queue"=w289) -> ("error out"=w283:errorcluster, "dup Message Queue"=w285:refnum<queue>)  [unwired: 6 in]
        n130 = call-poly "Enqueue Message.vi"("error in (no error)"=w283, "Message Data"=0 ("DISTANCE X 2"), "Message"="Goto_Y", "Message Queue"=w285) -> ("error out"=w280:errorcluster, "dup Message Queue"=w281:refnum<queue>)  [unwired: 6 in]
        n131 = call-poly "Enqueue Message.vi"("error in (no error)"=w280, "Message"="Rotate", "Message Queue"=w281) -> ("error out"=w279:errorcluster)  [unwired: 7 in, 1 out]
      }
      frame "Move_XY" {
        (unwired) 0.0 ("Numeric Control")
        # "run the table"
        # "iterate through matrix"
        n132 = local read "Y array"() -> (w303:dbl[])
        n133 = local read "X array"() -> (w304:dbl[])
        n134 = local read "Iteration"() -> (w296:u32)
        n135 = Index Array(array=w304, index=w296) -> (element=w300:dbl)
        n136 = Index Array(array=w303, index=w296) -> (element=w299:dbl)
        n137 = call-poly "Enqueue Message.vi"("Message Data"=w300, "Message"="Goto_X", "Message Queue"=w297) -> ("error out"=w295:errorcluster, "dup Message Queue"=w298:refnum<queue>)  [unwired: 7 in]
        n138 = call-poly "Enqueue Message.vi"("error in (no error)"=w295, "Message Data"=w299, "Message"="Goto_Y", "Message Queue"=w298) -> ("error out"=w293:errorcluster)  [unwired: 6 in, 1 out]
        n139 = call-poly "Enqueue Message.vi"("error in (no error)"=w293, "Message"="Rotate", "Message Queue"=w294) -> ()  [unwired: 7 in, 2 out]
        n140 = Merge Errors(w305) -> (w306:errorcluster)
      }
      frame "Rotate" {
        n141 = Bundle By Name(cluster=T8 {"revolution"=-1, "angle"=60000} ("Cluster"), "revolution"="revolution", "angle"=0) -> (w311:T8)
        n142 = Negate(x="revolution") -> (-x=w308:i32)
        n143 = local write "revolution"(w308) -> ()
        n144 = call-poly "Enqueue Message.vi"("Message Data"=w311, "Message"="Rotate", "Message Queue"=w313) -> ()  [unwired: 7 in, 2 out]
      }
      frame "increment" {
        n145 = local read "Iteration"() -> (w318:u32)
        n146 = Increment(x=w318) -> (x+1=w317:u32)
        n147 = local write "Iteration"(w317) -> ()
      }
      frame "Exit" {
        # "Stop the VI"
        # "Release the message queue reference"
        # "#CodeNeeded - Add any required cleanup code here. Note that if 'Exit' was called as a result of an error, an error dialog will be displayed. Add any custom error handling for an 'Exit' condition here as well."
        # "Exit - Exit the application."
        n148 = Variant To Data(type=errorcluster {"status"=FALSE, "code"=0, "source"=""} ("error constant"), Variant=w324) -> (data=w325:errorcluster)  [unwired: 1 in, 1 out]
        n149 = call <vilib>:"Simple Error Handler.vi"("error in (no error)"=w325) -> ()  [unwired: 4 in, 5 out]
        n150 = call "Fire User Event - Stop.vi"("User Event - Stop"=w329) -> ("error out"=w328:errorcluster)  [unwired: 10 in]
        n151 = Release Queue(queue=w334, error in (no error)=w327) -> (error out=w331:errorcluster)  [unwired: 1 in, 2 out]
        n152 = call-poly "Enqueue Message.vi"("Message"="Exit", "Message Queue"=w323) -> ("error out"=w321:errorcluster)  [unwired: 8 in, 1 out]
        n153 = Merge Errors(w321, w328, w331) -> (w330:errorcluster)
      }
      frame Default {
        # "'Default' case only runs if there is a message that isn't defined in any of the other cases.  Output a programming error."
        n154 = xnode "Error Ring"("parameter 0"=w335) -> ("error out"=w336:errorcluster)
      }
    }
    n155 = call "Error Handler - Message Handling Loop.vi"("error in (no error)"=w213, "Message Queue"=w215) -> ("dup error in"=w214:errorcluster)  [unwired: 8 in, 1 out]
  }
  n156 = local write "connected"(FALSE ("connected")) -> ()
  n157 = property on="connect" class="Bool"("Strings [4]"=string[] ["Connect"]) -> ()  [unwired: 2 in, 2 out]
  n158 = Unregister For Events(event registration refnum=w13, error in=w11) -> (error out=w14:errorcluster)
  n159 = Merge Errors(w14, w17) -> (w15:errorcluster)
  n160 = call "Destroy User Event - Stop.vi"("error in (no error)"=w15, "User Event - Stop"=w9) -> ("error out"=w5:errorcluster)  [unwired: 9 in]
  n161 = disable-structure shown="RUN_TIME_ENGINE==True" {
    disable-tunnel: w5 -> [_ _]
    frame condition #0 (active) {
    }
    frame condition #1 {
      # "Call Quit LabVIEW if running as a built application."
      n162 = Quit LabVIEW() -> ()  [unwired: 1 in]
    }
  }
  n163 = local read "connected"() -> (w4:bool)
  n164 = case shown="False" w4 {
    tunnel: w5 -> [_ _]
    frame False {
      n165 = local read "System Index"() -> (w345:u32)
      n166 = call <vilib>:"SA_CloseSystem.vi"("systemIndex"=w345) -> ()  [unwired: 10 in, 1 out]
    }
    frame True {
    }
  }
